vi "check_simulator.vi"(2 "error in":errorcluster, 3 "simx in":T1={"Config"={"Trajectory"={"Number of frames"=0, "Frame number"=0, "Trajectory"=""}, "Weather"={"id"=""}}, "Connections"={"Simulator Connection"=refnum, "server_ip"="127.0.0.1", "Port"=0, "Sensor connections"=[]}, "Map"={"lanes"={"x"=[], "y"=[], "z"=[]}, "StartPosition"={"start_points"={"locations"=[], "rotations"=[], "type"=[]}, "StartRotation"=[], "StartLocation"=[]}, "Draw Map Size"={"Width"=0, "Height"=0}, "DrawArea"={"min_Y"=0.0, "min_X"=0.0, "Scale X"=0.0, "Scale Y"=0.0}, "Map"=bytes[0], "Map Geojson"=""}}) -> (0 "error out":errorcluster, 1 "Connected":bool)   [LabVIEW 2025]
doc: "Check if the simulator is open and running. If it is not running then it will stop running the client."
uses:
  controls/simx_connection.ctl
  controls/config.ctl
  controls/trajectory.ctl
  controls/weather.ctl
  controls/connections.ctl
  controls/start_points.ctl
  <vilib>/Utility/miscctls.llb/LVBoundsTypeDef.ctl
panel:
  out "Editor error":string
  out "Editor Output":string
  out "Vehicle.exe output":string
  out "Vehicle.exe error":string
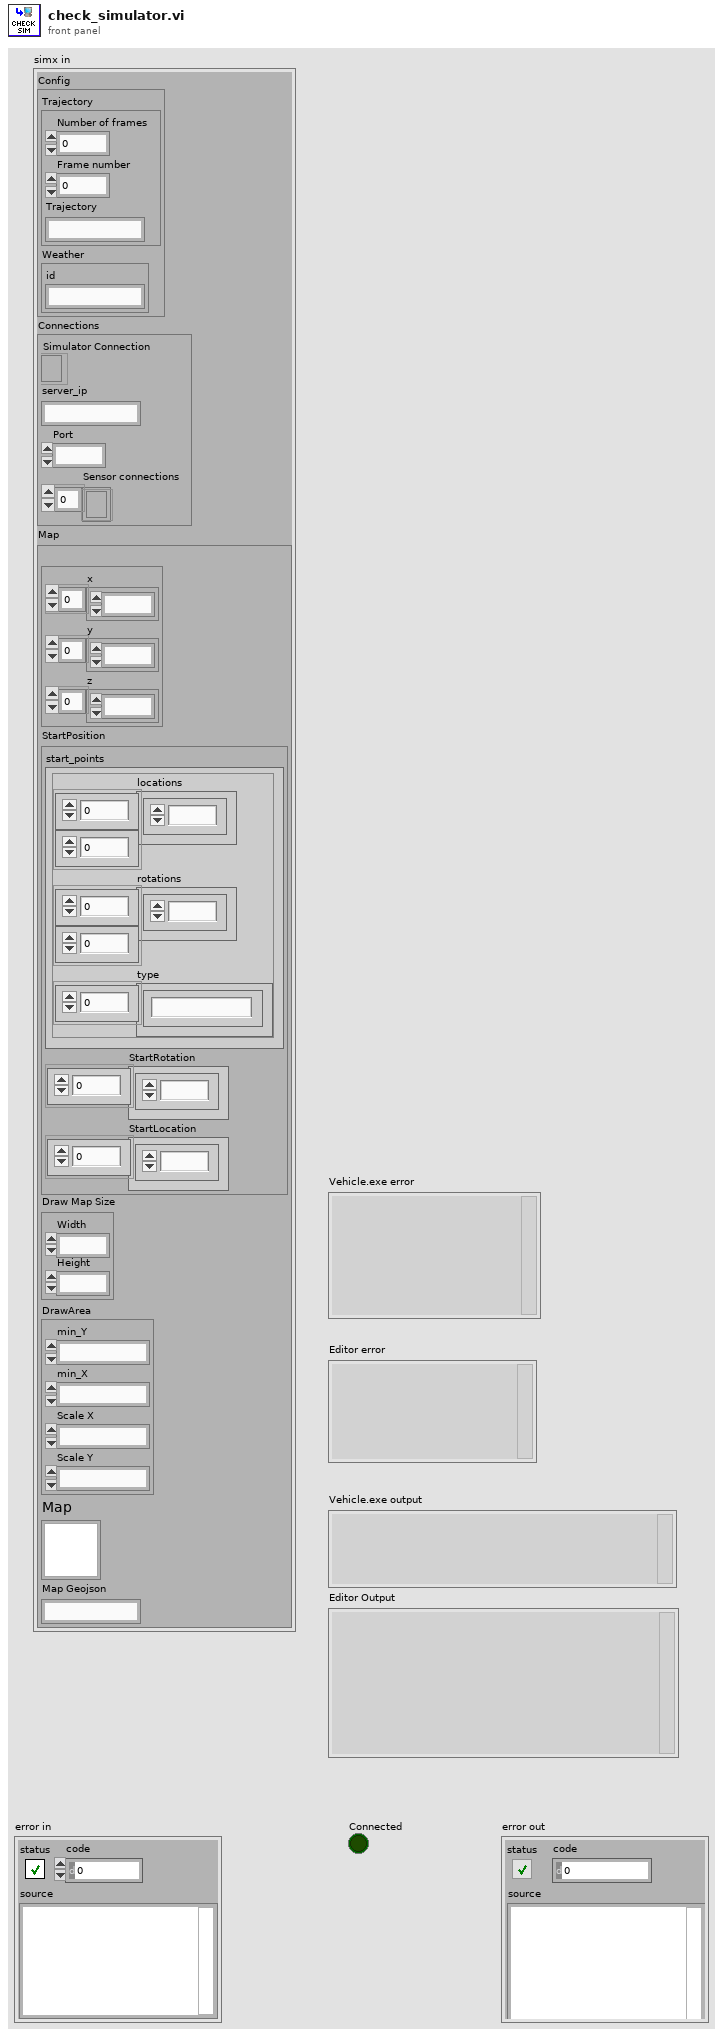
[diagram p1: front panel]
types:
  T1 = typedef "simx_connection.ctl" = cluster{"Config":T2, "Connections":T5, "Map":cluster{"lanes":cluster{"x":dbl[], "y":dbl[], "z":dbl[]}, "StartPosition":cluster{"start_points":T6, "StartRotation":dbl[], "StartLocation":dbl[]}, "Draw Map Size":T7, "DrawArea":cluster{"min_Y":dbl, "min_X":dbl, "Scale X":dbl, "Scale Y":dbl}, "Map":picture, "Map Geojson":string}}
  T2 = typedef "config.ctl" = cluster{"Trajectory":T3, "Weather":T4}
  T3 = typedef "trajectory.ctl" = cluster{"Number of frames":i32, "Frame number":i32, "Trajectory":string}
  T4 = typedef "weather.ctl" = cluster{"id":string}
  T5 = typedef "connections.ctl" = cluster{"Simulator Connection":refnum<k5>, "server_ip":string, "Port":i32, "Sensor connections":refnum<k5>[]}
  T6 = typedef "start_points.ctl" = cluster{"locations":dbl[][], "rotations":dbl[][], "type":string[]}
  T7 = typedef "LVBoundsTypeDef.ctl" = cluster{"Width":u32, "Height":u32}
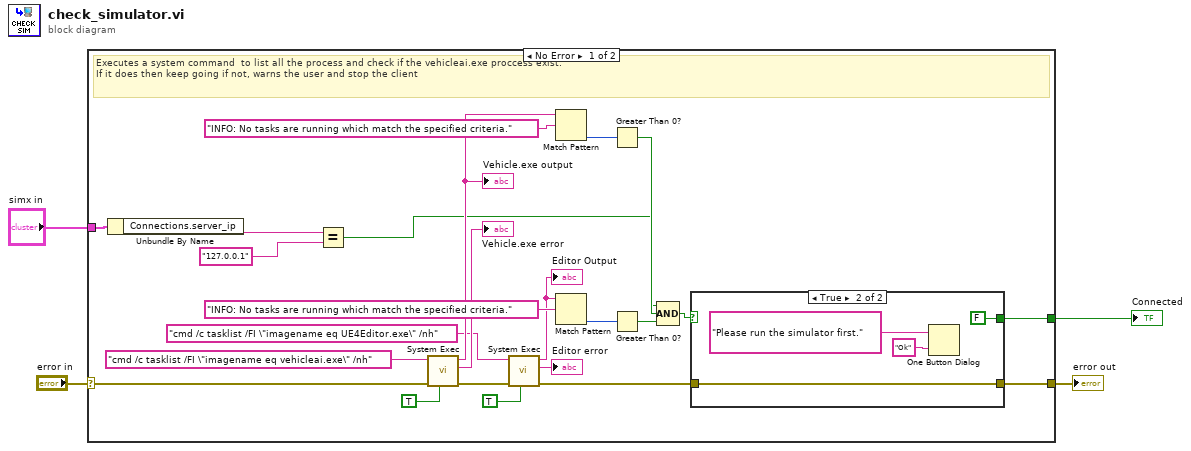
[diagram p0: block diagram]
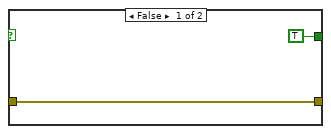
[diagram p2: hidden frame]
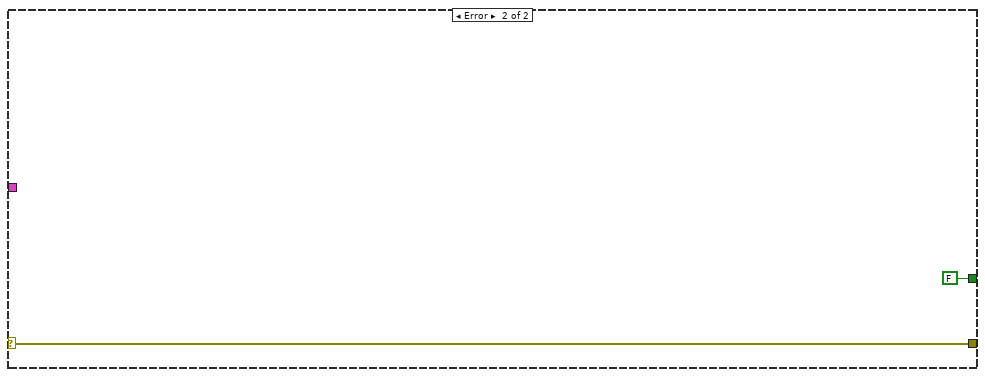
[diagram p3: hidden frame]
diagram:
  n1 = case shown="No Error" "error in" {
    selector: "error in" -> [w27 w36]
    tunnel: [w26 w36] -> w3
    tunnel: [w10 FALSE ("Connected")] -> w2
    tunnel: "simx in" -> [w8 _]
    frame No Error {
      # "Executes a system command  to list all the process and check if the vehicleai.exe proccess exist. \nIf it does then keep going if not, warns the user and stop the client"
      n2 = Unbundle By Name(w8) -> ("Connections.server_ip"=w7:string)
      n3 = Equal?(x=w7, y="127.0.0.1") -> (x = y?=w5:bool)
      n4 = call <vilib>:"System Exec.vi"("run minimized? (F)"=TRUE, "error in (no error)"=w27, "command line"="cmd /c tasklist /FI \"imagename eq vehicleai.exe\" /nh") -> ("error out"=w15:errorcluster, "standard error"=→"Vehicle.exe error":string, "standard output"=w23:string)  [unwired: 5 in, 1 out]
      "Vehicle.exe output" <- w23
      n5 = call <vilib>:"System Exec.vi"("run minimized? (F)"=TRUE, "error in (no error)"=w15, "command line"="cmd /c tasklist /FI \"imagename eq UE4Editor.exe\" /nh") -> ("error out"=w9:errorcluster, "standard error"=→"Editor error":string, "standard output"=w19:string)  [unwired: 5 in, 1 out]
      "Editor Output" <- w19
      n6 = Match Pattern(string=w23, regular expression="INFO: No tasks are running which match the specified criteria." ("x")) -> (offset past match=w21:i32)  [unwired: 1 in, 3 out]
      n7 = Match Pattern(string=w19, regular expression="INFO: No tasks are running which match the specified criteria." ("x")) -> (offset past match=w14:i32)  [unwired: 1 in, 3 out]
      n8 = Greater Than 0?(x=w21) -> (x > 0?=w12:bool)
      n9 = Greater Than 0?(x=w14) -> (x > 0?=w13:bool)
      n10 = Compound Arithmetic op=AND(w5, w12, w13) -> (w11:bool)
      n11 = case shown="True" w11 {
        tunnel: [w29 w31] -> w26
        tunnel: [TRUE ("Connected") FALSE ("Connected")] -> w10
        tunnel: w9 -> [w29 w31]
        frame False {
        }
        frame True {
          n12 = One Button Dialog(message="Please run the simulator first.", button name ("OK")="Ok") -> ()  [unwired: 1 out]
        }
      }
    }
    frame Error {
    }
  }
  "error out" <- w3
  "Connected" <- w2
